vi "VIP_Pre-Uninstall Custom Action 2021.vi"(10 "Variant":variant) -> (0 "error out":errorcluster)   [LabVIEW 2021]
uses:
  <vilib>/Utility/sysdir.llb/System Directory Type.ctl
  <userlib>/_OpenG.lib/file/file.llb/Build Path - Traditional__ogtk.vi
  <userlib>/_OpenG.lib/lvzip/lvzip.llb/subVI/ZLIB Extract All Files To Dir (Path)__ogtk.vi
  <resource>/dialog/lvconfig.llb/LV Config Read String.vi
  <vilib>/regexp/Match Regular Expression.xnode
  <userlib>/_OpenG.lib/file/file.llb/openg_file.lvlib
panel:
  # "pre uninstall"
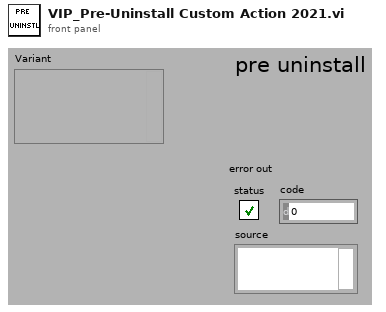
[diagram p1: front panel]
types:
  T1 = typedef "System Directory Type.ctl" = i32
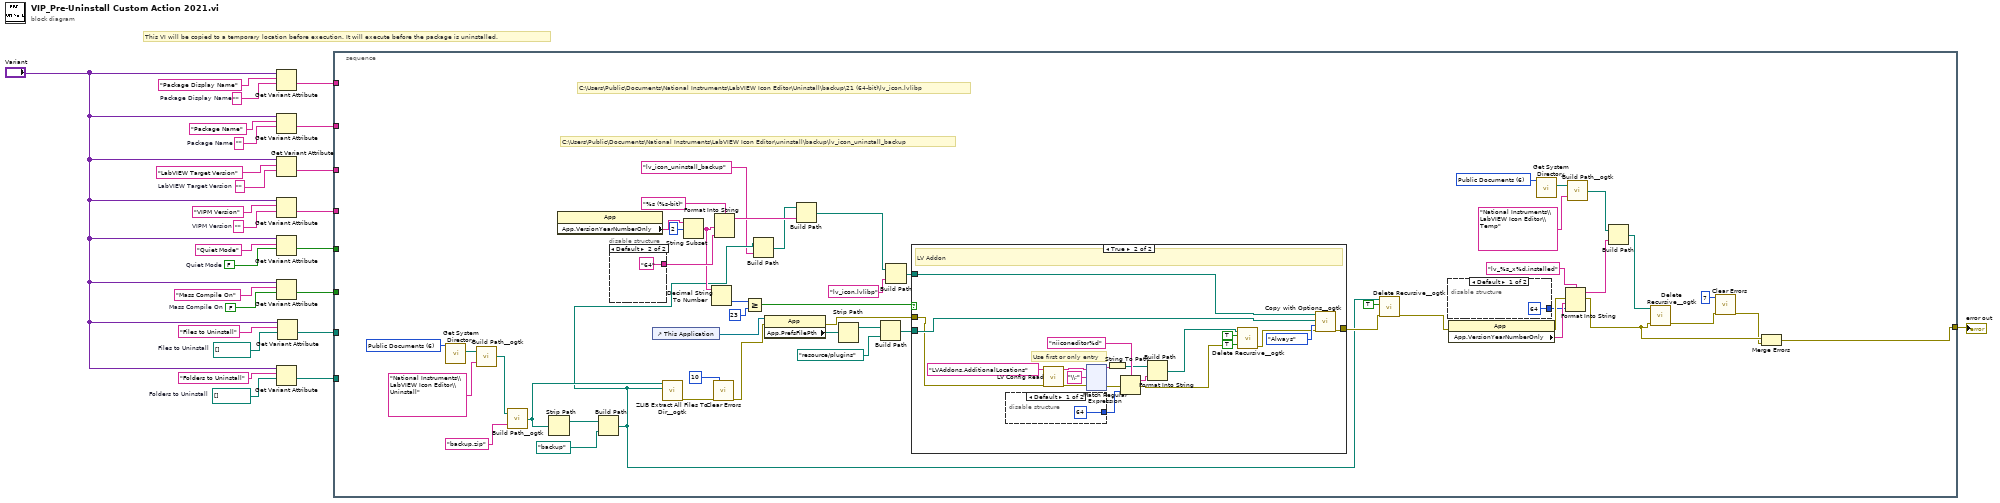
[diagram p0: block diagram]
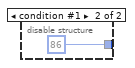
[diagram p2: hidden frame]
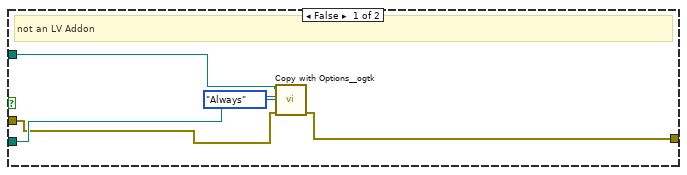
[diagram p3: hidden frame]
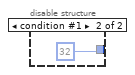
[diagram p4: hidden frame]
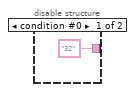
[diagram p5: hidden frame]
diagram:
  w11 = path[] []  # Folders to Uninstall
  w14 = path[] []  # Files to Uninstall
  w15 = FALSE  # Mass Compile On
  w16 = ""  # Package Display Name
  w17 = FALSE  # Quiet Mode
  w20 = ""  # VIPM Version
  w22 = ""  # LabVIEW Target Version
  w24 = ""  # Package Name
  # "This VI will be copied to a temporary location before execution. It will execute before the package is uninstalled."
  n1 = Get Variant Attribute(Variant="Variant", name="Package Display Name", default value (empty Variant)=w16) -> (value=w9:string)  [unwired: 1 in, 3 out]
  n2 = Get Variant Attribute(Variant="Variant", name="Package Name", default value (empty Variant)=w24) -> (value=w8:string)  [unwired: 1 in, 3 out]
  n3 = Get Variant Attribute(Variant="Variant", name="LabVIEW Target Version", default value (empty Variant)=w22) -> (value=w7:string)  [unwired: 1 in, 3 out]
  n4 = Get Variant Attribute(Variant="Variant", name="VIPM Version", default value (empty Variant)=w20) -> (value=w6:string)  [unwired: 1 in, 3 out]
  n5 = Get Variant Attribute(Variant="Variant", name="Quiet Mode", default value (empty Variant)=w17) -> (value=w5:bool)  [unwired: 1 in, 3 out]
  n6 = Get Variant Attribute(Variant="Variant", name="Mass Compile On", default value (empty Variant)=w15) -> (value=w4:bool)  [unwired: 1 in, 3 out]
  n7 = Get Variant Attribute(Variant="Variant", name="Folders to Uninstall", default value (empty Variant)=w11) -> (value=w2:path[])  [unwired: 1 in, 3 out]
  n8 = Get Variant Attribute(Variant="Variant", name="Files to Uninstall", default value (empty Variant)=w14) -> (value=w3:path[])  [unwired: 1 in, 3 out]
  n9 = stacked-sequence {
    tunnel: w9 -> [_]
    tunnel: w8 -> [_]
    tunnel: w7 -> [_]
    tunnel: w6 -> [_]
    tunnel: w5 -> [_]
    tunnel: w4 -> [_]
    tunnel: w3 -> [_]
    tunnel: w2 -> [_]
    tunnel: [w27] -> w1
    frame #0 {
      w43 = T1 6 items=["User Home"=0, "User Desktop"=1, "User Documents"=2, "User Application Data"=3, "User Preferences"=4, "User Temporary"=5, "Public Documents"=6, "Public Application Data"=7, "Public Preferences"=8, "Public Cache"=13, "System Core Libraries"=9, "System Installed Libraries"=10, "Application Files"=11, "Boot Volume Root"=12] ("system directory type")
      w58 = T1 6 items=["User Home"=0, "User Desktop"=1, "User Documents"=2, "User Application Data"=3, "User Preferences"=4, "User Temporary"=5, "Public Documents"=6, "Public Application Data"=7, "Public Preferences"=8, "Public Cache"=13, "System Core Libraries"=9, "System Installed Libraries"=10, "Application Files"=11, "Boot Volume Root"=12] ("system directory type")
      # "C:\\Users\\Public\\Documents\\National Instruments\\LabVIEW Icon Editor\\uninstall\\backup\\lv_icon_uninstall_backup"
      # "C:\\Users\\Public\\Documents\\National Instruments\\LabVIEW Icon Editor\\Uninstall\\backup\\21 (64-bit)\\lv_icon.lvlibp"
      n10 = call <vilib>:"Get System Directory.vi"("system directory type"=w58) -> ("system directory"=w57:path)  [unwired: 10 in]
      n11 = call-poly <userlib>:"Build Path__ogtk.vi"("name or relative path"="National Instruments\\LabVIEW Icon Editor\\Uninstall", "base path"=w57) -> ("appended path"=w54:path)
      n12 = call-poly <userlib>:"Build Path__ogtk.vi"("name or relative path"="backup.zip", "base path"=w54) -> ("appended path"=w49:path)
      n13 = Strip Path(path=w49) -> (stripped path=w53:path)  [unwired: 1 out]
      n14 = property class="App"() -> ("App.VersionYearNumberOnly"=w62:string)  [unwired: 2 in, 2 out]
      n15 = Build Path(base path=w53, name or relative path=path "backup") -> (appended path=w35:path)
      n16 = disable-structure shown="Default" {
        disable-tunnel: ["32" "64"] -> w75
        frame condition #0 {
        }
        frame condition #1 (active) {
        }
      }
      n17 = control-ref of="This Application"() -> (w59:refnum<vi>)
      n18 = call-poly <userlib>:"ZLIB Extract All Files To Dir__ogtk.vi"("destination directory (archive name without ending)"=w35, "archive name (file dialog)"=w49) -> ("error out"=w38:errorcluster)  [unwired: 7 in, 2 out]
      n19 = String Subset(string=w62, offset (0)=2) -> (substring=w61:string)  [unwired: 1 in]
      n20 = Decimal String To Number(string=w61) -> (number=w73:i32)  [unwired: 2 in, 1 out]
      n21 = call <vilib>:"Clear Errors.vi"("error in (no error)"=w38, "specific error code to clear (0: all)"=10) -> ("error out"=w37:errorcluster)  [unwired: 4 in, 1 out]
      n22 = Format Into String(format string="%s (%s-bit)", w61, w75) -> (resulting string=w65:string)  [unwired: 2 in, 1 out]
      n23 = Greater Or Equal?(x=w73, y=23) -> (x >= y?=w67:bool)
      n24 = Build Path(base path=w35, name or relative path="lv_icon_uninstall_backup" ("resulting string")) -> (appended path=w34:path)
      n25 = property class="App"(reference=w59, error in=w37) -> (error out=w64:errorcluster, "App.PrefsFilePth"=w74:path)  [unwired: 1 out]
      n26 = Build Path(base path=w34, name or relative path=w65) -> (appended path=w60:path)
      n27 = Strip Path(path=w74) -> (stripped path=w71:path)  [unwired: 1 out]
      n28 = Build Path(base path=w71, name or relative path=path "resource/plugins") -> (appended path=w69:path)
      n29 = Build Path(base path=w60, name or relative path="lv_icon.lvlibp" ("resulting string")) -> (appended path=w66:path)
      n30 = case shown="True" w67 {
        tunnel: [w79 w103] -> w48
        tunnel: w69 -> [w81 w100]
        tunnel: w66 -> [w82 w101]
        tunnel: w64 -> [w80 w89]
        frame False {
          # "not an LV Addon"
          n31 = call <userlib>:"Copy with Options__ogtk.vi"("error in (no error)"=w80, "Replace Mode (Never)"=enum16{"Never", "Always", "If Newer"}."Always", "target path"=w81, "source path"=w82) -> ("error out"=w79:errorcluster)  [unwired: 6 in, 1 out]
        }
        frame True {
          # "Use first or only entry"
          # "LV Addon"
          n32 = disable-structure shown="Default" {
            disable-tunnel: [64 ("code") 32 ("code")] -> w94
            frame condition #0 (active) {
            }
            frame condition #1 {
            }
          }
          n33 = call-poly <resource>:"LV Config Read.vi"("error in"=w89, "key"="LVAddons.AdditionalLocations") -> ("error out"=w95:errorcluster, "value"=w93:string)  [unwired: 3 in, 1 out]
          n34 = xnode "Match Regular Expression"("input string"=w93, "regular expression"="\\;", "error in"=w95) -> ("before match"=w87:string, "error out"=w96:errorcluster)  [unwired: 3 in, 3 out]
          n35 = String To Path(string=w87) -> (path=w86:path)
          n36 = Format Into String(format string="niiconeditor%d", error in=w96, w94) -> (resulting string=w85:string, error out=w88:errorcluster)  [unwired: 1 in]
          n37 = Build Path(base path=w86, name or relative path=w85) -> (appended path=w84:path)
          n38 = call <userlib>:"Delete Recursive__ogtk.vi"("error in (no error)"=w88, "Ignore Read-Only? (FALSE)"=TRUE, "Recursive? (FALSE)"=TRUE, "Path"=w84) -> ("error out"=w99:errorcluster)  [unwired: 6 in, 1 out]
          n39 = call <userlib>:"Copy with Options__ogtk.vi"("error in (no error)"=w99, "Replace Mode (Never)"=enum16{"Never", "Always", "If Newer"}."Always", "target path"=w100, "source path"=w101) -> ("error out"=w103:errorcluster)  [unwired: 6 in, 1 out]
        }
      }
      n40 = call <userlib>:"Delete Recursive__ogtk.vi"("error in (no error)"=w48, "Recursive? (FALSE)"=TRUE, "Path"=w35) -> ("error out"=w47:errorcluster)  [unwired: 7 in, 1 out]
      n41 = disable-structure shown="Default" {
        disable-tunnel: [64 ("code") 86 ("code")] -> w41
        frame condition #0 (active) {
        }
        frame condition #1 {
        }
      }
      n42 = property class="App"(error in=w47) -> (error out=w50:errorcluster, "App.VersionYearNumberOnly"=w42:string)  [unwired: 1 in, 1 out]
      n43 = call <vilib>:"Get System Directory.vi"("system directory type"=w43) -> ("system directory"=w44:path)  [unwired: 10 in]
      n44 = Format Into String(format string="lv_%s_x%d.installed", error in=w50, w42, w41) -> (resulting string=w40:string, error out=w29:errorcluster)  [unwired: 1 in]
      n45 = call-poly <userlib>:"Build Path__ogtk.vi"("name or relative path"="National Instruments\\LabVIEW Icon Editor\\Temp", "base path"=w44) -> ("appended path"=w39:path)
      n46 = Build Path(base path=w39, name or relative path=w40) -> (appended path=w32:path)
      n47 = call <userlib>:"Delete Recursive__ogtk.vi"("error in (no error)"=w29, "Path"=w32) -> ("error out"=w31:errorcluster)  [unwired: 8 in, 1 out]
      n48 = call <vilib>:"Clear Errors.vi"("error in (no error)"=w31, "specific error code to clear (0: all)"=7) -> ("error out"=w28:errorcluster)  [unwired: 4 in, 1 out]
      n49 = Merge Errors(w29, w28) -> (w27:errorcluster)
    }
  }
  "error out" <- w1
